vi "Autotune PID Cascade.vi"(7 "Unit Address (1)":i16=1, 8 "error in (no error)":errorcluster {"code" format="%.0x"}, 9 "Cascade Outer Loop (0: Tune Off)":u16(ring) items=["Tune Off", "Outer Loop PID Set 1", "Outer Loop PID Set 2", "Outer Loop PID Set 3", "Outer Loop PID Set 4", "Outer Loop PID Set 5"], 10 "Cascade Inner Loop (0: Tune Off)":u16(ring) items=["Tune Off", "Inner Loop PID Set 1", "Inner Loop PID Set 2", "Inner Loop PID Set 3", "Inner Loop PID Set 4", "Inner Loop PID Set 5"], 11 "VISA resource name":refnum<visa-resource-name>) -> (0 "error out":errorcluster {"code" format="%.0x"}, 3 "VISA resource name out":refnum<visa-resource-name>)   [LabVIEW 2010]
doc: "This VI configures autotune PID cascade."
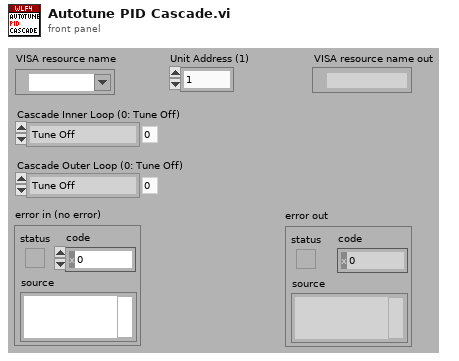
[diagram p1: front panel]
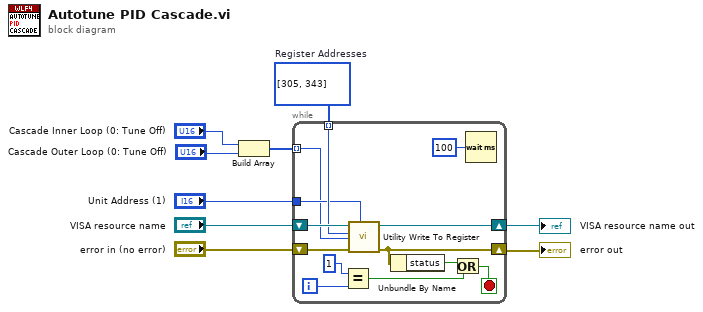
[diagram p0: block diagram]
diagram:
  w7 = i32[] [305, 343]  # Register Addresses
  n1 = Build Array("Cascade Inner Loop (0: Tune Off)", "Cascade Outer Loop (0: Tune Off)") -> (w5:u16[])
  n2 = while {
    shift-right: [w20] -> w2
    shift-left: "VISA resource name" -> [w22]
    shift-right: [w18] -> w1
    shift-left: "error in (no error)" -> [w21]
    tunnel: w7 -> [w12] mode=indexing
    tunnel: "Unit Address (1)" -> [w11]
    tunnel: w5 -> [w10] mode=indexing
    i -> [w14]
    stop <- w16 stop-if-true
    n3 = Equal?(x=1, y=w14) -> (x = y?=w13:bool)
    n4 = call "Utility Write To Register.vi"("Unit Address (1)"=w11, "error in (no error)"=w21, "Data (0)"=w10, "Register Address (0)"=w12, "VISA resource name"=w22) -> ("error out"=w18:errorcluster, "VISA resource name out"=w20:refnum<visa-resource-name>)  [unwired: 5 in]
    n5 = Unbundle By Name(w18) -> ("status"=w17:bool)
    n6 = Or(x=w17, y=w13) -> (x .or. y?=w16:bool)
    n7 = Wait (ms)(milliseconds to wait=u32 100) -> ()  [unwired: 1 out]
  }
  "error out" <- w1
  "VISA resource name out" <- w2
